vi "Play add to cluster.vi"() -> ()   [LabVIEW 2014]
panel:
  in  "Add on":bool
  out "Output cluster":T1
  in  "Input cluster":T2
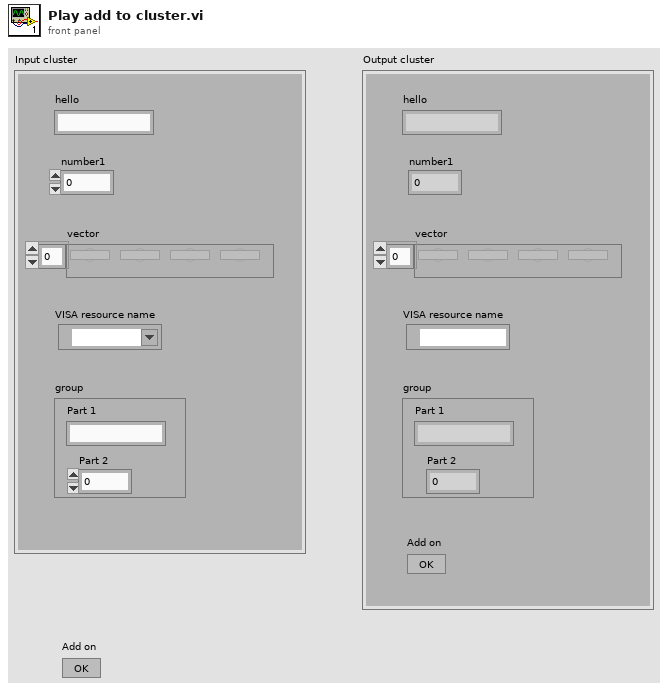
[diagram p1: front panel]
types:
  T1 = cluster{"hello":string, "number1":dbl, "vector":bool[], "VISA resource name":refnum<visa-resource-name>, "group":cluster{"Part 1":string, "Part 2":dbl}, "Add on":bool}
  T2 = cluster{"hello":string, "number1":dbl, "vector":bool[], "VISA resource name":refnum<visa-resource-name>, "group":cluster{"Part 1":string, "Part 2":dbl}}
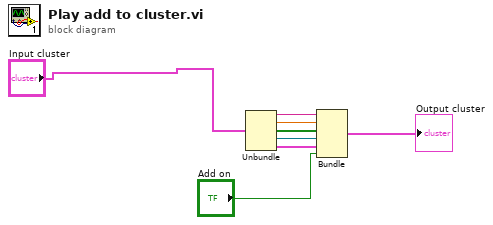
[diagram p0: block diagram]
diagram:
  n1 = Unbundle("Input cluster") -> ("hello"=w8:string, "number1"=w7:dbl, "vector"=w6:bool[], "VISA resource name"=w5:refnum<visa-resource-name>, "group"=w4:cluster{"Part 1":string, "Part 2":dbl})
  n2 = Bundle("hello"=w8, "number1"=w7, "vector"=w6, "VISA resource name"=w5, "group"=w4, "Add on"="Add on") -> (→"Output cluster":T1)  [unwired: 1 in]
